vi "ep_Decimation Factor Calculation.vi"(9 "filter for frequency measurement":T1={"enable filter? (T)"=TRUE, "passband edge frequency [Hz]"=0.0, "passband ripple [dB]"=0.1, "stopband edge frequency [Hz]"=0.0, "stopband attenuation [dB]"=60.0}, 10 "maximum frequency [Hz]":dbl, 11 "fs [Hz]":dbl) -> (2 "decimation factor":i32, 3 "fs after decimation [Hz]":dbl, 5 "dup fs [Hz]":dbl)   [LabVIEW 2013, in "NI_EP_Power Measurement.lvlib"]
uses:
  <vilib>/addons/Electrical Power/Power Measurement/NI_EP_Power Measurement.lvlib
  <vilib>/addons/Electrical Power/Power Measurement/subVIs/ep_Filter Design.ctl
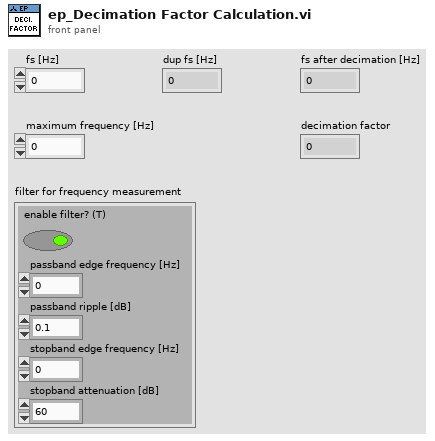
[diagram p1: front panel]
types:
  T1 = typedef "NI_EP_Power Measurement.lvlib/ep_Filter Design.ctl" = cluster{"enable filter? (T)":bool, "passband edge frequency [Hz]":dbl, "passband ripple [dB]":dbl, "stopband edge frequency [Hz]":dbl, "stopband attenuation [dB]":dbl}
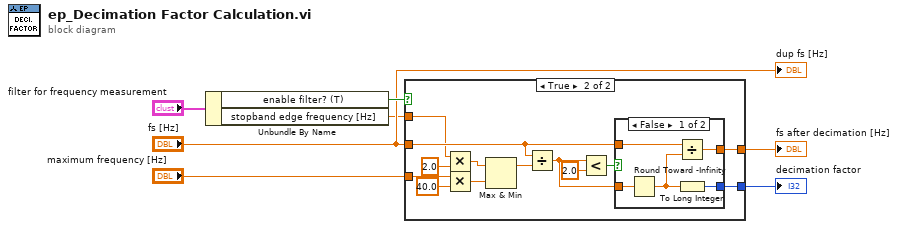
[diagram p0: block diagram]
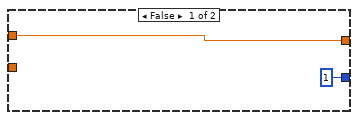
[diagram p2: hidden frame]
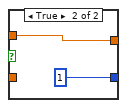
[diagram p3: hidden frame]
diagram:
  n1 = Unbundle By Name("filter for frequency measurement") -> ("enable filter? (T)"=w3:bool, "stopband edge frequency [Hz]"=w1:dbl)
  n2 = case shown="True" w3 {
    tunnel: "maximum frequency [Hz]" -> [_ w18]
    tunnel: [1 ("decimation factor") w17] -> w6
    tunnel: [w9 w16] -> w5
    tunnel: "fs [Hz]" -> [w9 w15]
    tunnel: w1 -> [_ w13]
    frame False {
    }
    frame True {
      n3 = Multiply(x=w13, y=2.0) -> (x*y=w11:dbl)
      n4 = Multiply(x=w18, y=40.0) -> (x*y=w12:dbl)
      n5 = Max & Min(x=w11, y=w12) -> (max(x,y)=w10:dbl)  [unwired: 1 out]
      n6 = Divide(x=w15, y=w10) -> (x/y=w19:dbl)
      n7 = Less?(x=w19, y=2.0) -> (x < y?=w20:bool)
      n8 = case shown="False" w20 {
        tunnel: w15 -> [w26 w28]
        tunnel: [w25 1 ("decimation factor")] -> w17
        tunnel: [w23 w28] -> w16
        tunnel: w19 -> [w27 _]
        frame False {
          n9 = Round Toward -Infinity(1:w27) -> (0:w24:dbl)
          n10 = Divide(x=w26, y=w24) -> (x/y=w23:dbl)
          n11 = To Long Integer(number=w24) -> (32bit integer=w25:i32)
        }
        frame True {
        }
      }
    }
  }
  "fs after decimation [Hz]" <- w5
  "decimation factor" <- w6
  "dup fs [Hz]" <- "fs [Hz]"
